vi "Source Function.vi"(7 "Function (Current)":enum32{"Current", "Voltage"}(ring), 8 "error in (no error)":errorcluster, 9 "Channel (Channel A)":T1, 10 "Node In":string, 11 "VISA resource name":refnum<visa-resource-name>) -> (0 "error out":errorcluster, 2 "Node Out":string, 3 "VISA resource name out":refnum<visa-resource-name>, 4 "Command String":string)   [LabVIEW 2018, in "Keithley 2600 Series.lvlib"]
doc: "This VI sets the source function of the selected SMU channel. Source function may be Current or Voltage.\n\n<b>Functions and Attributes Used</b>\nsmuX.source.func"
uses:
  Keithley 2600 Series.lvlib
  Channel.ctl
  GlobalVariables.vi
panel:
  # "(c) 2008 Keithley Instruments, Inc.  ALL RIGHTS RESERVED."
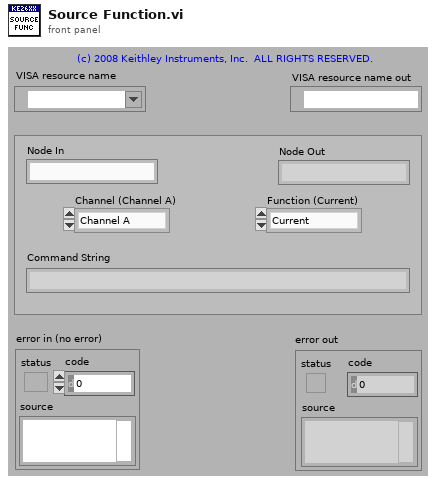
[diagram p1: front panel]
types:
  T1 = typedef "Keithley 2600 Series.lvlib/Channel.ctl" = enum32{"Channel A", "Channel B"}
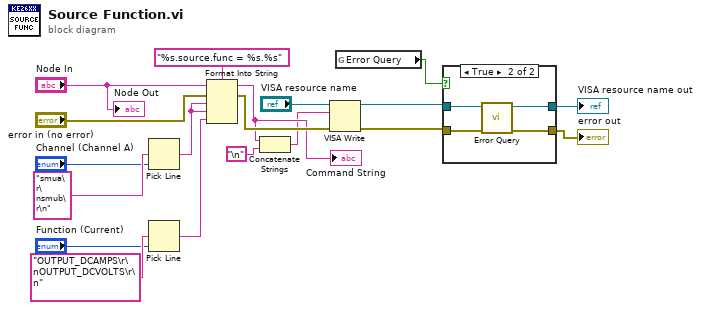
[diagram p0: block diagram]
diagram:
  n1 = Pick Line(multi-line string="smua\r\nsmub\r\n" ("options"), line index="Channel (Channel A)") -> (output string=w10:string)  [unwired: 1 out]
  n2 = Pick Line(multi-line string="OUTPUT_DCAMPS\r\nOUTPUT_DCVOLTS\r\n" ("options"), line index="Function (Current)") -> (output string=w9:string)  [unwired: 1 out]
  n3 = Format Into String(format string="%s.source.func = %s.%s", initial string="Node In", error in="error in (no error)", w10, w10, w9) -> (resulting string=w2:string, error out=w6:errorcluster)
  "Command String" <- w2
  n4 = Concatenate Strings(w2, "\n") -> (w1:string)
  n5 = VISA Write(VISA resource name="VISA resource name", write buffer=w1, error in (no error)=w6) -> (VISA resource name out=w4:refnum<visa-resource-name>, error out=w5:errorcluster)  [unwired: 1 out]
  n6 = global read "GlobalVariables.vi" "Error Query"() -> (w15:bool)
  n7 = case shown="True" w15 {
    tunnel: w4 -> [w21 w25]
    tunnel: w5 -> [w20 w24]
    tunnel: [w21 w23] -> w14
    tunnel: [w20 w22] -> w13
    frame False {
    }
    frame True {
      n8 = call "Error Query.vi"("error in (no error)"=w24, "VISA resource name"=w25) -> ("error out"=w22:errorcluster, "VISA resource name out"=w23:refnum<visa-resource-name>)  [unwired: 8 out]
    }
  }
  "VISA resource name out" <- w14
  "error out" <- w13
  "Node Out" <- "Node In"
